vi "Stepper3D.vi"() -> ()   [LabVIEW 2014, in "stepper3D.lvlib"]
uses:
  stepper3D.lvlib
  <vilib>/Instr/_visa.llb/VISA Configure Serial Port (Instr).vi
  <vilib>/event_ctls.llb/eventvkey.ctl
  Enums/BoundaryStatus.ctl
panel:
  out "status":T2
  in  "M18":bool
  in  "speed":string="100"
  out "Initialized":bool
  in  "move to position":dbl[](array[numeric])
  in  "set current position":dbl[](array[numeric])
  in  "Move to Position":bool
  in  "Set Current Position":bool
  out "result":string
  in  "stop":bool
  in  "send":bool
  in  "command":string
  in  "VISA resource name":refnum<visa-resource-name>="COM8"
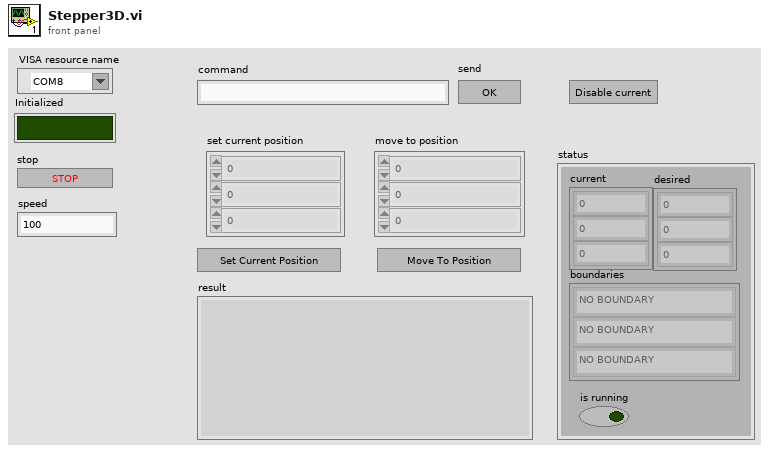
[diagram p1: front panel]
types:
  T1 = typedef "stepper3D.lvlib/BoundaryStatus.ctl" = enum16{"NO BOUNDARY", "OUT OF LEFT", "OUT OF RIGHT"}
  T2 = cluster{"desired":dbl[], "current":dbl[], "boundaries":T1[], "is running":bool}
  T3 = typedef "eventvkey.ctl" = enum16{"ASCII", "Enter", "Return", "Shift", "Ctrl", "Alt", "Cmd", "Opt", "Caps", "NumLock", "Clear", "Break", "Up", "Down", "Left", "Right", "Insert", "Delete", "Home", "End", "PageUp", "PageDown", "Escape", "Help", "Pause", "ScrollLock", "F1", "F2", "F3", "F4", "F5", "F6", "F7", "F8", "F9", "F10", "F11", "F12", "F13", "F14", "F15", "F16", "F17", "F18", "F19", "F20", "F21", "F22", "F23", "F24", "Play", "VolumeUp", "VolumeDown", "Mute", "Two Byte Char"}
  T4 = typedef "stepper3D.lvlib/CurrentStatus.ctl" = cluster{"desired":dbl[], "current":dbl[], "boundaries":T1[], "is running":bool}
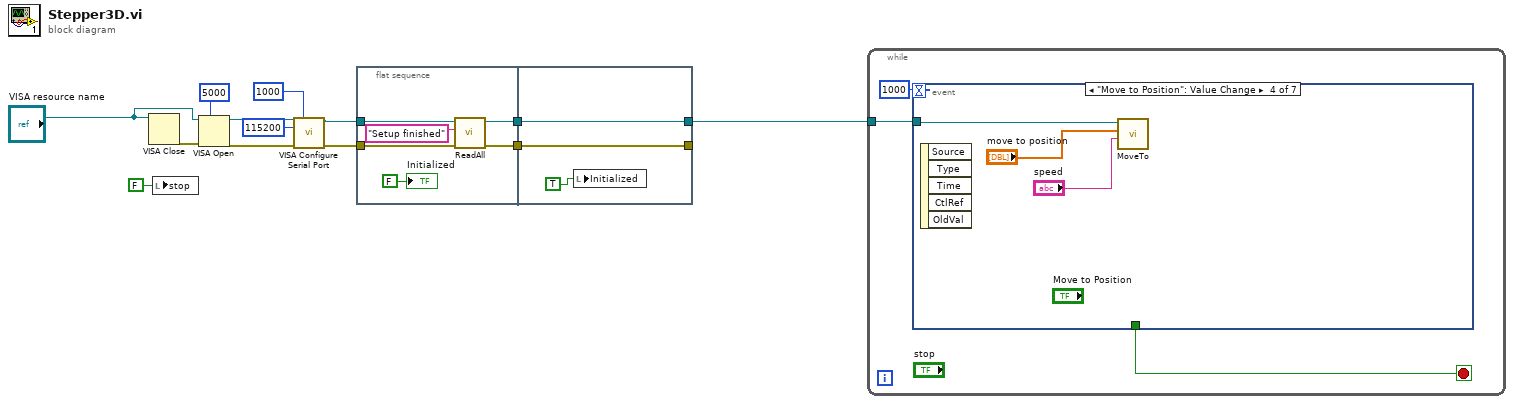
[diagram p0: block diagram]
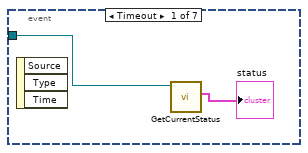
[diagram p2: hidden frame]
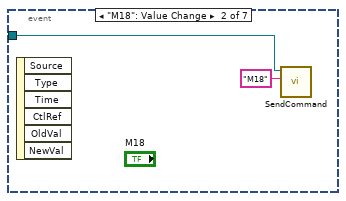
[diagram p3: hidden frame]
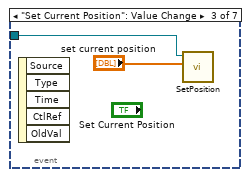
[diagram p4: hidden frame]
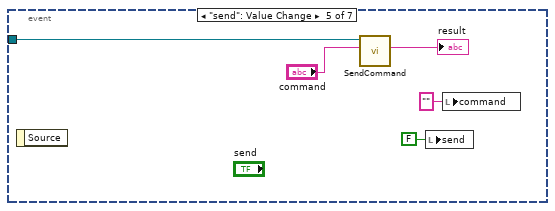
[diagram p5: hidden frame]
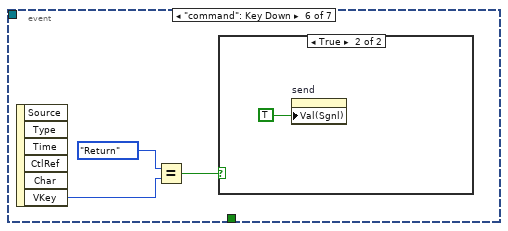
[diagram p6: hidden frame]
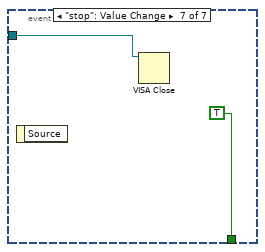
[diagram p8: hidden frame]
diagram:
  n1 = VISA Close(VISA resource name="VISA resource name") -> (error out=w7:errorcluster)  [unwired: 1 in]
  n2 = local write "stop"(FALSE ("stop")) -> ()
  n3 = VISA Open(timeout (0)=u32 5000 ("VISA Open timeout (0)"), error in (no error)=w7, VISA resource name="VISA resource name") -> (VISA resource name=w12:refnum<visa-resource-name>, error out=w10:errorcluster)  [unwired: 2 in]
  n4 = call-poly "VISA Configure Serial Port"("VISA resource name"=w12, "timeout (10sec)"=u32 1000, "baud rate (9600)"=u32 115200, "error in (no error)"=w10) -> ("VISA resource name out"=w9:refnum<visa-resource-name>, "error out"=w8:errorcluster)  [unwired: 10 in]
  n5 = flat-sequence {
    tunnel: [w19] -> w3
    tunnel: [w16] -> w2
    tunnel: w9 -> [w18]
    tunnel: w8 -> [w17]
    tunnel: [w21] -> _
    tunnel: [w22] -> w4
    tunnel: w3 -> [w22]
    tunnel: w2 -> [w21]
    frame #0 {
      n6 = call "ReadAll.vi"("error in (no error)"=w17, "value"="Setup finished", "VISA resource in"=w18) -> ("error out"=w16:errorcluster, "VISA resource out"=w19:refnum<visa-resource-name>)  [unwired: 5 in, 2 out]
      "Initialized" <- FALSE ("Initialized")
    }
    frame #1 {
      n7 = local write "Initialized"(TRUE ("Initialized")) -> ()
    }
  }
  n8 = while {
    tunnel: w4 -> [w25]
    stop <- w23 stop-if-true
    n9 = event shown="[3] \"Move to Position\": Value Change" {
      selector: _ -> [_ _ _ _ _ _ _]
      dyn-events: _ -> [_ _ _ _ _ _ _]
      timeout: 1000 ("Numeric") -> [_ _ _ _ _ _ _]
      tunnel: w25 -> [w27 w29 w30 w34 w39 _ w44]
      tunnel: [_ _ _ _ _ _ TRUE] -> w23
      event Timeout {
        n10 = event-data() -> ()  [unwired: 1 in, 3 out]
        n11 = call "GetCurrentStatus.vi"("VISA Refnum in"=w27) -> ("status"=→"status":T4)  [unwired: 8 in, 2 out]
      }
      event "M18": Value Change {
        n12 = event-data() -> ()  [unwired: 1 in, 6 out]
        n13 = call "SendCommand.vi"("command"="M18", "VISA Refnum in"=w29) -> ()  [unwired: 7 in, 3 out]
      }
      event "Set Current Position": Value Change {
        n14 = event-data() -> ()  [unwired: 1 in, 5 out]
        n15 = call "SetPosition.vi"("positions"="set current position", "VISA Refnum in"=w30) -> ()  [unwired: 8 in, 2 out]
      }
      event "Move to Position": Value Change {
        n16 = event-data() -> ()  [unwired: 1 in, 5 out]
        n17 = call "MoveTo.vi"("speed"="speed", "positions"="move to position", "VISA Refnum in"=w34) -> ()  [unwired: 7 in, 2 out]
      }
      event "send": Value Change {
        n18 = event-data() -> ()  [unwired: 1 in, 1 out]
        n19 = call "SendCommand.vi"("command"="command", "VISA Refnum in"=w39) -> ("result"=→"result":string)  [unwired: 7 in, 2 out]
        n20 = local write "send"(FALSE ("send")) -> ()
        n21 = local write "command"("" ("command")) -> ()
      }
      event "command": Key Down {
        n22 = event-data() -> ("VKey"=w41:T3)  [unwired: 1 in, 5 out]
        n23 = Equal?(x=eventvkey."Return" ("VKey"), y=w41) -> (x = y?=w40:bool)
        n24 = case shown="True" w40 {
          frame False {
          }
          frame True {
            n25 = property on="send" class="Bool (strict)"("Val(Sgnl)"=TRUE) -> ()  [unwired: 2 in, 2 out]
          }
        }
      }
      event "stop": Value Change {
        n26 = event-data() -> ()  [unwired: 1 in, 1 out]
        n27 = VISA Close(VISA resource name=w44) -> ()  [unwired: 1 in, 1 out]
      }
    }
  }
